vi "control motorv2.vi"() -> ()   [LabVIEW 2013]
panel:
  out "status 3":bool
  out "code 3":i32
  out "code 2":i32
  out "status 2":bool
  in  "source":string
  in  "code":i32
  in  "status":bool
  out "current state":string
  in  "Up/Down,Stay":T1(ring)
  out "floor 1":dbl
  out "floor 3":dbl
  out "floor 2":dbl
  in  "stop":bool
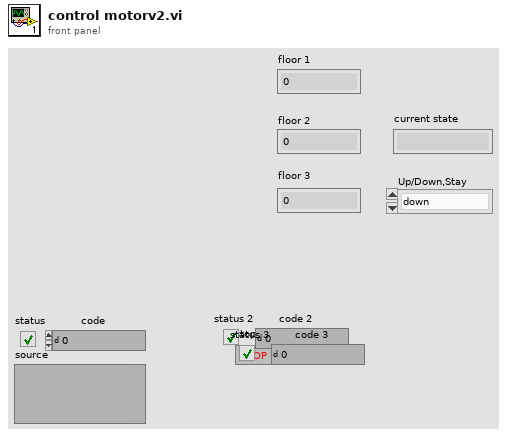
[diagram p1: front panel]
types:
  T1 = enum16{"down", "stay", "up", "1st to 3rd", "3rd to 1st"}
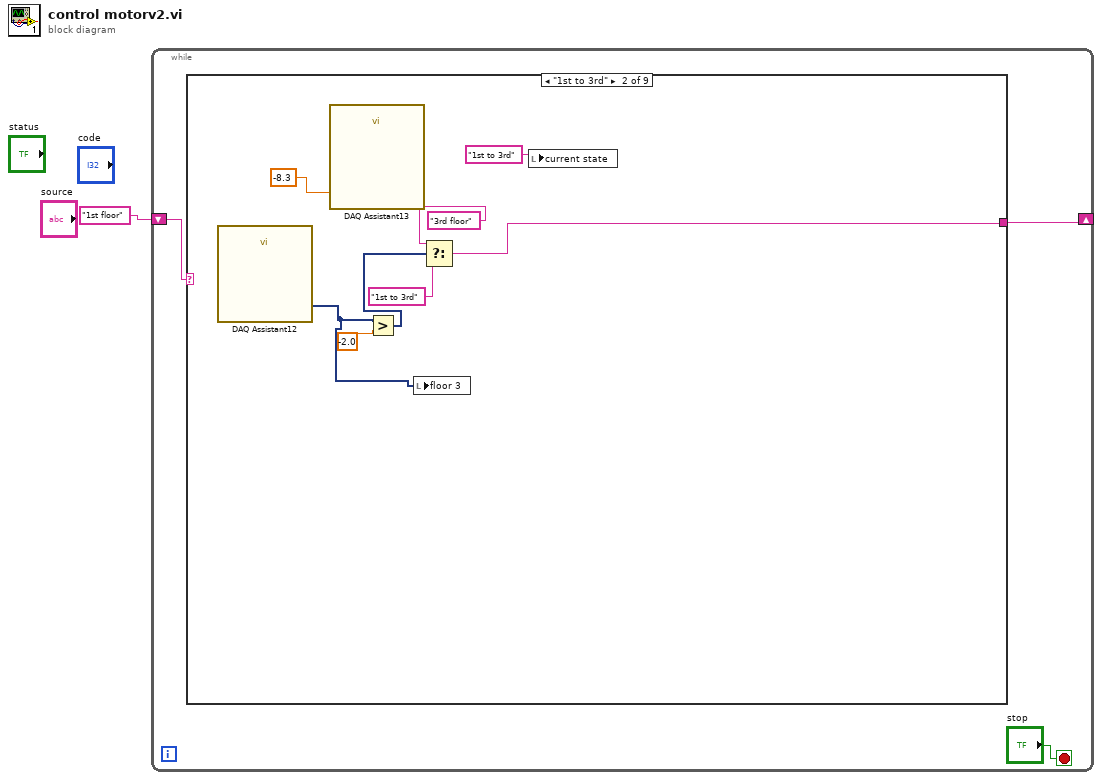
[diagram p0: block diagram]
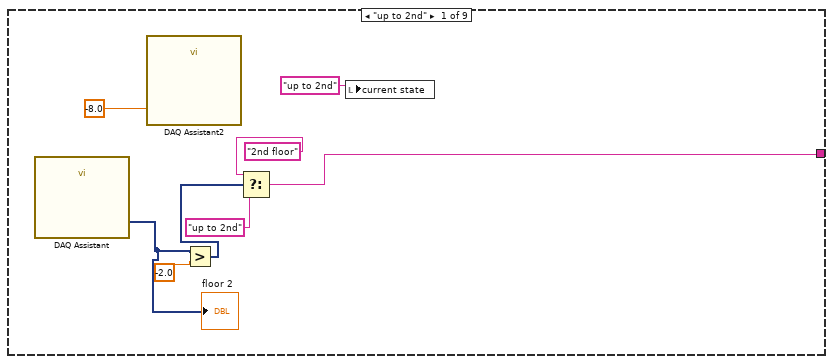
[diagram p2: hidden frame]
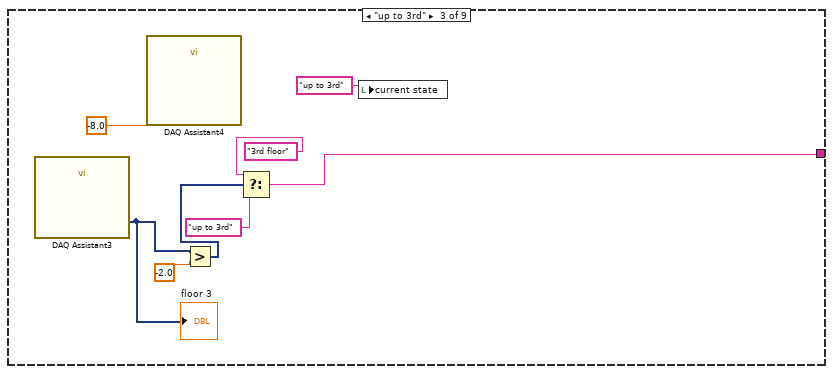
[diagram p3: hidden frame]
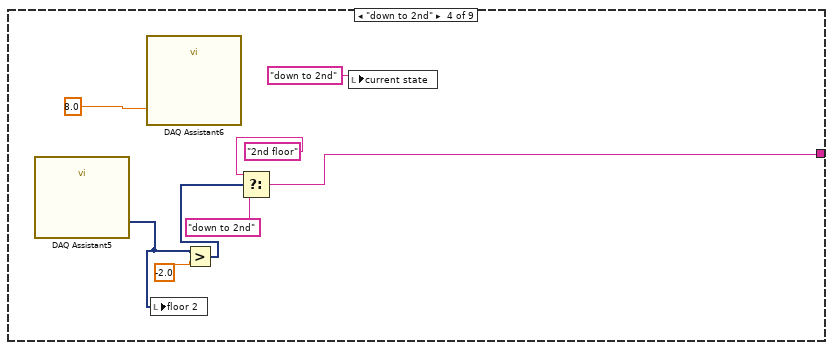
[diagram p4: hidden frame]
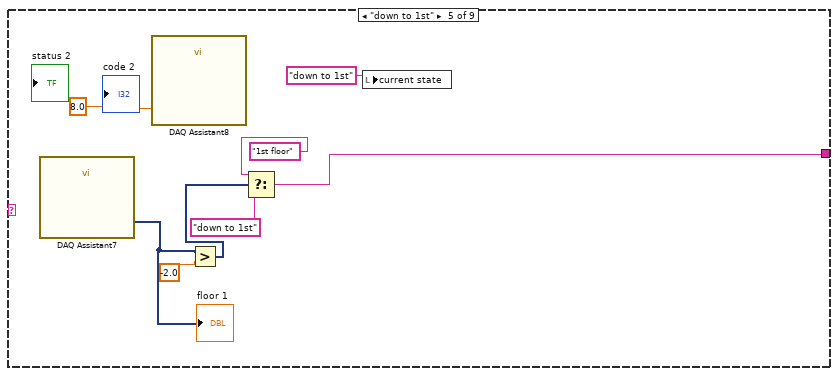
[diagram p5: hidden frame]
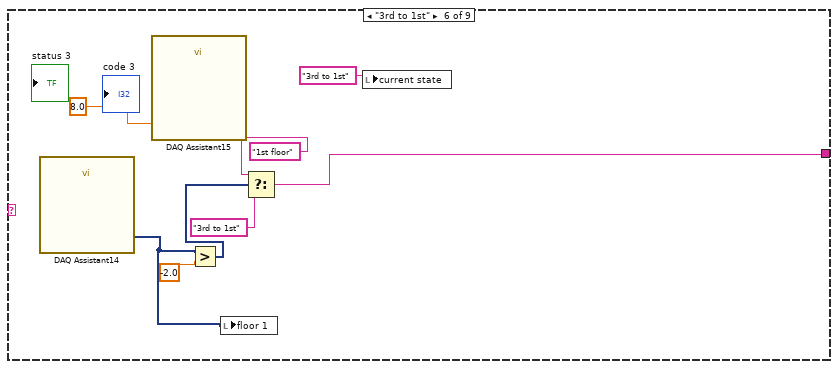
[diagram p6: hidden frame]
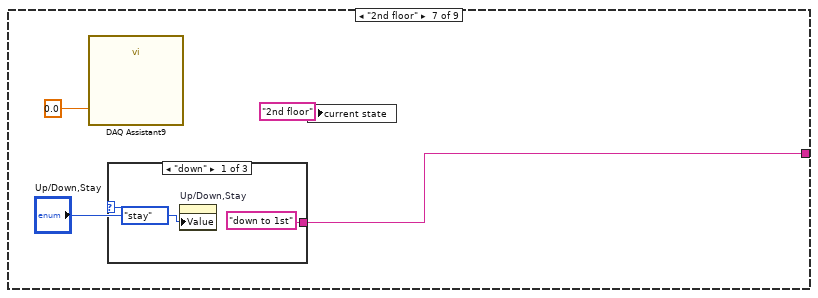
[diagram p7: hidden frame]
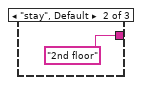
[diagram p8: hidden frame]
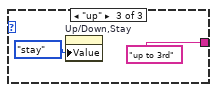
[diagram p9: hidden frame]
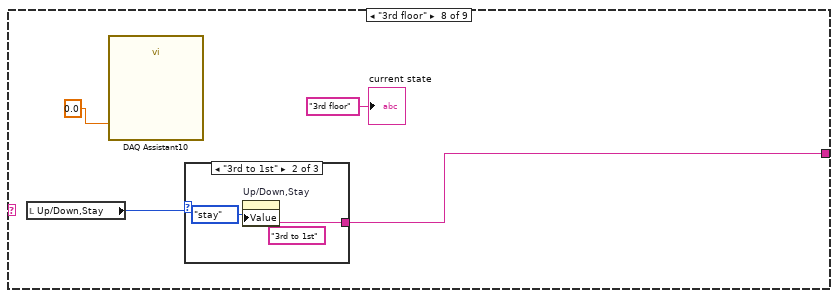
[diagram p10: hidden frame]
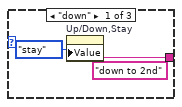
[diagram p11: hidden frame]
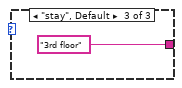
[diagram p12: hidden frame]
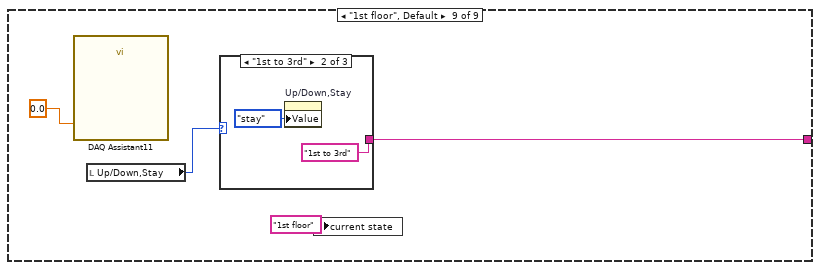
[diagram p13: hidden frame]
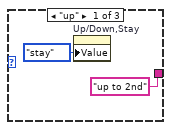
[diagram p14: hidden frame]
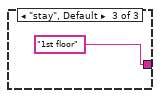
[diagram p15: hidden frame]
diagram:
  n1 = while {
    shift-right: [w3] -> _
    shift-left: "1st floor" -> [w4]
    stop <- "stop" stop-if-true
    n2 = case shown="\"1st to 3rd\"" w4 {
      tunnel: [w11 w19 w26 w34 w42 w50 w54 w64 w74] -> w3
      frame "up to 2nd" {
        n3 = call "DAQ Assistant"() -> ("data"=w8:dynamicdata)  [unwired: 17 in, 2 out]
        "floor 2" <- w8
        n4 = call "DAQ Assistant2"("data"=-8.0) -> ()  [unwired: 17 in, 2 out]
        n5 = Greater?(x=w8, y=-2.0) -> (0:w5:dynamicdata)
        n6 = Select(t="2nd floor", s=w5, f="up to 2nd") -> (s? t:f=w11:string)
        n7 = local write "current state"("up to 2nd" ("String")) -> ()
      }
      frame "1st to 3rd" {
        n8 = call "DAQ Assistant12"() -> ("data"=w13:dynamicdata)  [unwired: 17 in, 2 out]
        n9 = call "DAQ Assistant13"("data"=-8.3) -> ()  [unwired: 17 in, 2 out]
        n10 = Greater?(x=w13, y=-2.0) -> (0:w14:dynamicdata)
        n11 = local write "floor 3"(w13) -> ()
        n12 = Select(t="3rd floor", s=w14, f="1st to 3rd") -> (s? t:f=w19:string)
        n13 = local write "current state"("1st to 3rd" ("String")) -> ()
      }
      frame "up to 3rd" {
        n14 = call "DAQ Assistant3"() -> ("data"=w22:dynamicdata)  [unwired: 17 in, 2 out]
        "floor 3" <- w22
        n15 = call "DAQ Assistant4"("data"=-8.0) -> ()  [unwired: 17 in, 2 out]
        n16 = Greater?(x=w22, y=-2.0) -> (0:w21:dynamicdata)
        n17 = Select(t="3rd floor", s=w21, f="up to 3rd") -> (s? t:f=w26:string)
        n18 = local write "current state"("up to 3rd" ("String")) -> ()
      }
      frame "down to 2nd" {
        n19 = call "DAQ Assistant5"() -> ("data"=w30:dynamicdata)  [unwired: 17 in, 2 out]
        n20 = call "DAQ Assistant6"("data"=8.0) -> ()  [unwired: 17 in, 2 out]
        n21 = local write "floor 2"(w30) -> ()
        n22 = Greater?(x=w30, y=-2.0) -> (0:w29:dynamicdata)
        n23 = Select(t="2nd floor", s=w29, f="down to 2nd") -> (s? t:f=w34:string)
        n24 = local write "current state"("down to 2nd" ("String")) -> ()
      }
      frame "down to 1st" {
        n25 = call "DAQ Assistant7"() -> ("data"=w38:dynamicdata)  [unwired: 17 in, 2 out]
        "floor 1" <- w38
        n26 = call "DAQ Assistant8"("data"=8.0) -> ()  [unwired: 17 in, 2 out]
        n27 = Greater?(x=w38, y=-2.0) -> (0:w37:dynamicdata)
        n28 = Select(t="1st floor", s=w37, f="down to 1st") -> (s? t:f=w42:string)
        n29 = local write "current state"("down to 1st" ("String")) -> ()
      }
      frame "3rd to 1st" {
        n30 = call "DAQ Assistant14"() -> ("data"=w45:dynamicdata)  [unwired: 17 in, 2 out]
        n31 = call "DAQ Assistant15"("data"=8.0) -> ()  [unwired: 17 in, 2 out]
        n32 = Greater?(x=w45, y=-2.0) -> (0:w46:dynamicdata)
        n33 = local write "floor 1"(w45) -> ()
        n34 = Select(t="1st floor", s=w46, f="3rd to 1st") -> (s? t:f=w50:string)
        n35 = local write "current state"("3rd to 1st" ("String")) -> ()
      }
      frame "2nd floor" {
        n36 = call "DAQ Assistant9"("data"=0.0) -> ()  [unwired: 17 in, 2 out]
        n37 = case shown="\"down\"" "Up/Down,Stay" {
          tunnel: ["down to 1st" "2nd floor" "up to 3rd"] -> w54
          frame "down" {
            n38 = property on="Up/Down,Stay" class="Enum (strict)"("Value"=enum16{"down", "stay", "up"}."stay" ("Up/Down,Stay")) -> ()  [unwired: 2 in, 2 out]
          }
          frame "stay", Default {
          }
          frame "up" {
            n39 = property on="Up/Down,Stay" class="Enum (strict)"("Value"=enum16{"down", "stay", "up"}."stay" ("Up/Down,Stay")) -> ()  [unwired: 2 in, 2 out]
          }
        }
        n40 = local write "current state"("2nd floor" ("String")) -> ()
      }
      frame "3rd floor" {
        n41 = local read "Up/Down,Stay"() -> (w63:T1)
        n42 = call "DAQ Assistant10"("data"=0.0) -> ()  [unwired: 17 in, 2 out]
        n43 = case shown="\"3rd to 1st\"" w63 {
          tunnel: ["down to 2nd" "3rd to 1st" "3rd floor"] -> w64
          frame "down" {
            n44 = property on="Up/Down,Stay" class="Enum (strict)"("Value"=enum16{"down", "stay", "up"}."stay" ("Up/Down,Stay")) -> ()  [unwired: 2 in, 2 out]
          }
          frame "3rd to 1st" {
            n45 = property on="Up/Down,Stay" class="Enum (strict)"("Value"=enum16{"down", "stay", "up"}."stay" ("Up/Down,Stay")) -> ()  [unwired: 2 in, 2 out]
          }
          frame "stay", Default {
          }
        }
        "current state" <- "3rd floor" ("String")
      }
      frame "1st floor", Default {
        n46 = call "DAQ Assistant11"("data"=0.0) -> ()  [unwired: 17 in, 2 out]
        n47 = local read "Up/Down,Stay"() -> (w73:T1)
        n48 = case shown="\"1st to 3rd\"" w73 {
          tunnel: ["up to 2nd" "1st to 3rd" "1st floor"] -> w74
          frame "up" {
            n49 = property on="Up/Down,Stay" class="Enum (strict)"("Value"=enum16{"down", "stay", "up"}."stay" ("Up/Down,Stay")) -> ()  [unwired: 2 in, 2 out]
          }
          frame "1st to 3rd" {
            n50 = property on="Up/Down,Stay" class="Enum (strict)"("Value"=enum16{"down", "stay", "up"}."stay" ("Up/Down,Stay")) -> ()  [unwired: 2 in, 2 out]
          }
          frame "stay", Default {
          }
        }
        n51 = local write "current state"("1st floor" ("String")) -> ()
      }
    }
  }
